vi "write_delimiter.vi"() -> ()   [LabVIEW 2022 SP3]
uses:
  <vilib>/Utility/file.llb/Write Delimited Spreadsheet (string).vi
panel:
  in  "Array":cluster{"Value":dbl, "Message":string}[](array[cluster])
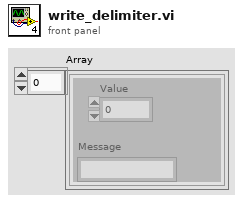
[diagram p1: front panel]
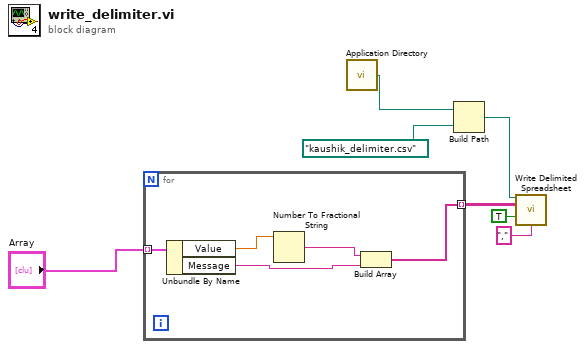
[diagram p0: block diagram]
diagram:
  n1 = for {
    tunnel: "Array" -> [w12] mode=indexing
    tunnel: [w8] -> w4 mode=indexing
    n2 = Unbundle By Name(w12) -> ("Value"=w11:dbl, "Message"=w10:string)
    n3 = Number To Fractional String(number=w11) -> (F-format string=w9:string)  [unwired: 3 in]
    n4 = Build Array(w9, w10) -> (w8:string[])
  }
  n5 = call <vilib>:"Application Directory.vi"() -> ("Application Directory"=w2:path)
  n6 = Build Path(base path=w2, name or relative path=path "kaushik_delimiter.csv") -> (appended path=w6:path)
  n7 = call-poly <vilib>:"Write Delimited Spreadsheet.vi"("file path (dialog if empty)"=w6, "2D data"=w4, "append to file? (new file:F)"=TRUE, "delimiter (\\t)"="," ("delimiter (\\t)")) -> ()  [unwired: 10 in, 2 out]
